vi "Calib_Inst_Type.vi"(1 "Input string":string) -> (0 "Instrument type":T2=enum."Pressure Transducer")   [LabVIEW 2011]
uses:
  Controls/Cal_Inst_type.ctl
panel:
  in  "Instrument type Orig":T1(ring)=enum."Cross wire velocity"
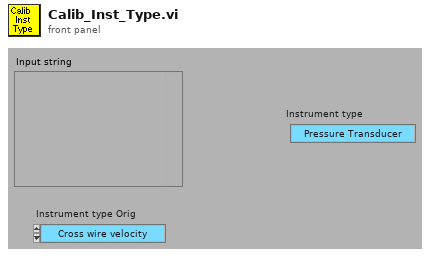
[diagram p1: front panel]
types:
  T1 = enum16{"Propeller anemometer", "Pressure Transducer", "Hot wire", "Cross wire velocity", "Cross wire angle", "Generic Instrument", "Fast FID", "Thermocouple", "Cold wire"}
  T2 = typedef "Cal_Inst_type.ctl" = enum16{"Propeller anemometer", "Pressure Transducer", "Hot wire", "Cross wire velocity", "Cross wire angle", "Generic Linear", "Generic Polynomial", "Generic BackPoly", "Fast FID", "Thermocouple", "Cold wire", "Pulsed Wire"}
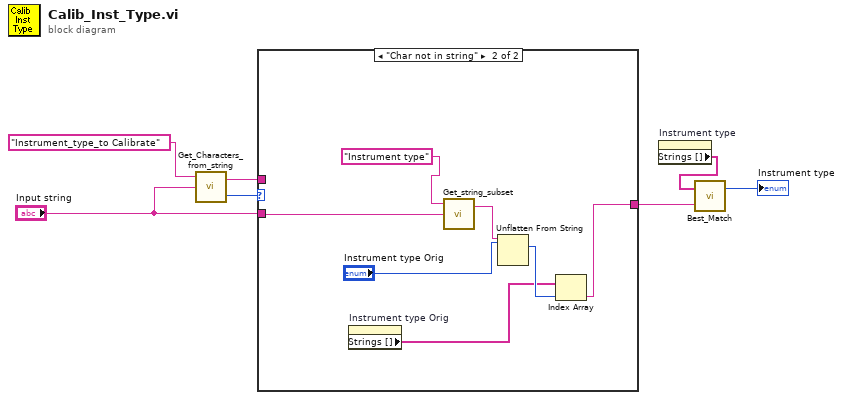
[diagram p0: block diagram]
diagram:
  n1 = call "Get_Characters_from_string.vi"("Input string"="Input string", "Variable name"="Instrument_type_to Calibrate") -> ("Status"=w6:enum16{"Char in string", "Char not in string"}, "Value"=w1:string)  [unwired: 1 in]
  n2 = case shown="\"Char not in string\"" w6 {
    tunnel: "Input string" -> [_ w13]
    tunnel: [w8 w9] -> w2
    tunnel: w1 -> [w8 _]
    frame "Char in string" {
    }
    frame "Char not in string" {
      n3 = property on="Instrument type Orig" class="Enum (strict)"() -> ("Strings []"=w10:string[])  [unwired: 2 in, 2 out]
      n4 = call "Get_string_subset.vi"("String to split"=w13, "File Label"="Instrument type") -> ("Output string"=w15:string)  [unwired: 2 in, 1 out]
      n5 = Unflatten From String(type="Instrument type Orig", binary string=w15) -> (value=w11:T1)  [unwired: 1 in, 4 out]
      n6 = Index Array(array=w10, index=w11) -> (element=w9:string)
    }
  }
  n7 = property on="Instrument type" class="Enum (strict)"() -> ("Strings []"=w3:string[])  [unwired: 2 in, 2 out]
  n8 = call "Best_Match.vi"("Input String"=w2, "String Options"=w3) -> ("index of element"=→"Instrument type":i32)  [unwired: 1 out]
